vi "Get DiliconMeasurement.vi"(8 "error in (no error)":errorcluster, 10 "Dilico Measurement Controls":T3 {"Wait time [ms]" max=26}, 11 "input cluster":T4={"Session_Control"="Sess_Control", "Session_Params"="Sess_Params", "Session_Actuals"="Sess_Actuals", "Session_Acknowledge"="Sess_Ack", "Session_H2_Sensor"="H2_Sensor_Session", "Session_DILICO_MeasurementRequest"="Session_DILICO_MeasurementRequest", "Session_DILICO_Voltages"="Session_DILICO_CELLVoltage"}) -> (0 "error out":errorcluster, 2 "CAN Frame Output":T1[](array[typedef]) {"payload" format="%x"; "timestamp" format="%<%.7X\n%x>T"; "type" items=["CAN Data"=0, "CAN Remote"=1, "CAN Bus Error"=2, "CAN 2.0 Data"=8, "CAN FD Data"=16, "CAN FD+BRS Data"=24, "J1939 Data"=192, "Delay"=224, "Log Trigger"=225, "Start Trigger"=226]; "identifier" format="%x"}, 3 "output cluster":T4={"Session_Control"="Session_Control", "Session_Params"="Session_Params", "Session_Actuals"="Session_Actuals", "Session_Acknowledge"="Session_Acknowledge", "Session_H2_Sensor"="H2_Sensor_Session", "Session_DILICO_MeasurementRequest"="Session_DILICO_MeasurementRequest", "Session_DILICO_Voltages"="Session_DILICO_CELLVoltage"})   [LabVIEW 2025, in "phlair-busch-can-bus.lvlib"]
uses:
  phlair-busch-can-bus.lvlib
  CAN Frame Sessions.ctl
  DilicoControls.ctl
  <vilib>/xnet/xnet.llb/XNET Frame CAN.ctl
  <vilib>/xnet/xnet.llb/XNET Frame Type CAN.ctl
  <vilib>/xnet/xnet.llb/XNET Write (Signal Single-point).vi
  <vilib>/xnet/xnet.llb/XNET Read (Frame CAN).vi
  <resource>/objmgr/xnet.rc
panel:
  out "Array 2":u32[](array[numeric])
  out "Array":dbl[](array[numeric])
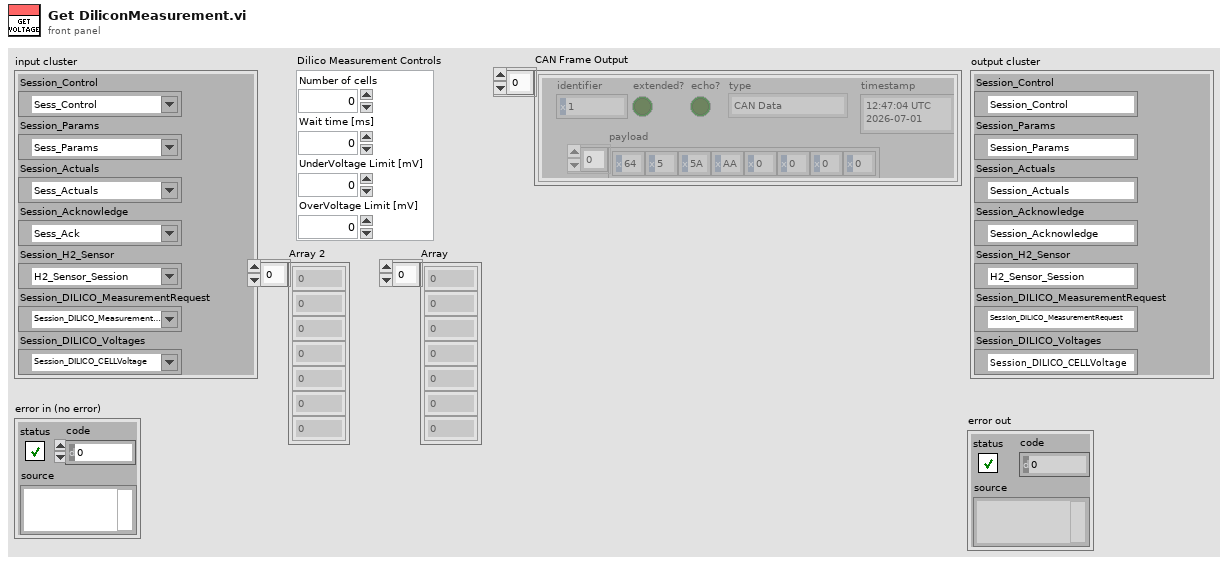
[diagram p1: front panel]
types:
  T1 = typedef "XNET Frame CAN.ctl" = cluster{"timestamp":timestamp, "payload":u8[], "identifier":u32, "type":T2, "extended?":bool, "echo?":bool}
  T2 = typedef "XNET Frame Type CAN.ctl" = u8
  T3 = typedef "phlair-busch-can-bus.lvlib/DilicoControls.ctl" = cluster{"Number of cells":u8, "Wait time [ms]":sgl, "UnderVoltage Limit [mV]":u16, "OverVoltage Limit [mV]":u16}
  T4 = typedef "phlair-busch-can-bus.lvlib/CAN Frame Sessions.ctl" = cluster{"Session_Control":refnum<k21>, "Session_Params":refnum<k21>, "Session_Actuals":refnum<k21>, "Session_Acknowledge":refnum<k21>, "Session_H2_Sensor":refnum<k21>, "Session_DILICO_MeasurementRequest":refnum<k21>, "Session_DILICO_Voltages":refnum<k21>}
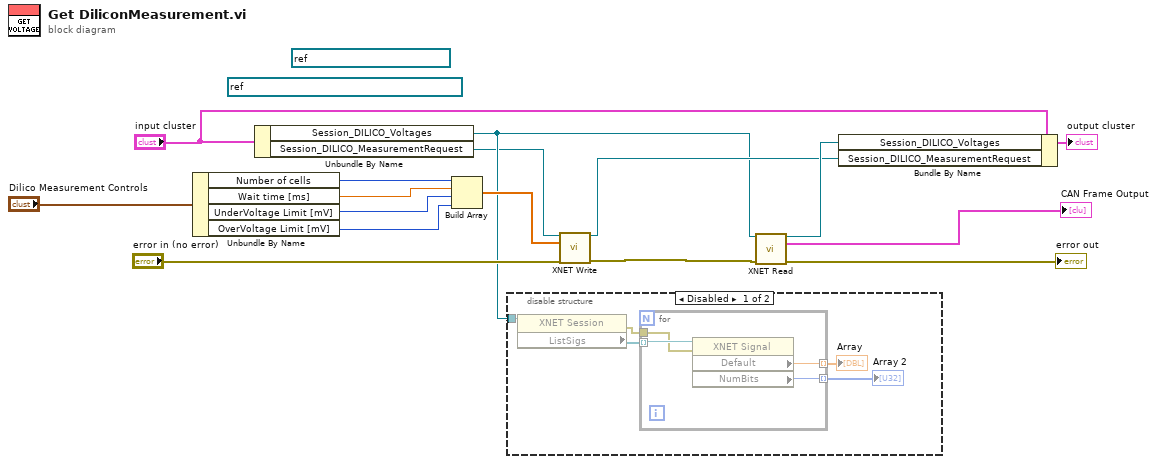
[diagram p0: block diagram]
diagram:
  (unwired) refnum<k21> "Session_DILOCO_MeasurementRequest" ("Session_DILICO_Voltages")
  (unwired) refnum<k21> "Session_DILICO_Voltages" ("Session_DILICO_Voltages")
  n1 = Unbundle By Name("Dilico Measurement Controls") -> ("Number of cells"=w8:u8, "Wait time [ms]"=w3:sgl, "UnderVoltage Limit [mV]"=w1:u16, "OverVoltage Limit [mV]"=w2:u16)
  n2 = Unbundle By Name("input cluster") -> ("Session_DILICO_Voltages"=w6:refnum<k21>, "Session_DILICO_MeasurementRequest"=w5:refnum<k21>)
  n3 = Build Array(w8, w3, w1, w2) -> (w10:sgl[])
  n4 = disable-structure shown="Disabled" {
    disable-tunnel: w6 -> [w17 _]
    frame Disabled {
      n5 = property class="XNET Session"(reference=w17) -> (error out=w18:errorcluster, "ListSigs"=w21:refnum<k21>[])  [unwired: 1 in, 1 out]
      n6 = for {
        tunnel: w21 -> [w25] mode=indexing
        tunnel: [w24] -> w20 mode=indexing
        tunnel: [w23] -> w19 mode=indexing
        tunnel: w18 -> [w22]
        n7 = property class="XNET Signal"(reference=w25, error in=w22) -> ("Default"=w24:dbl, "NumBits"=w23:u32)  [unwired: 2 out]
      }
      "Array" <- w20
      "Array 2" <- w19
    }
    frame Enabled {
    }
  }
  n8 = call-poly <vilib>:"XNET Write.vi"("session in"=w5, "data"=w10, "error in (no error)"="error in (no error)") -> ("session out"=w9:refnum<k21>, "error out"=w7:errorcluster)  [unwired: 11 in]
  n9 = call-poly <vilib>:"XNET Read.vi"("session in"=w6, "error in (no error)"=w7) -> ("session out"=w15:refnum<k21>, "data"=→"CAN Frame Output":T1[], "error out"=→"error out":errorcluster)  [unwired: 10 in, 1 out]
  n10 = Bundle By Name(cluster="input cluster", "Session_DILICO_Voltages"=w15, "Session_DILICO_MeasurementRequest"=w9) -> (→"output cluster":T4)
